vi "Specified_Channels_server.vi"(5 "Mode":T1, 6 "End time":dbl format="%.1f", 7 "Start time":dbl format="%.1f", 8 "Clients time":dbl, 9 "Requested channels":i32[](array[numeric])) -> (0 "Output array":dbl[][](array[numeric]) format="%.2f", 1 "Messages":string, 2 "Averaging Period":dbl[](array[numeric]) format="%.2f", 3 "Centre Times":dbl[](array[numeric]) format="%.1f", 4 "All Active Ch Names":string[](array[string]))   [LabVIEW 2021]
uses:
  ADAM Client/Sub VIs/ADAM Controls/Search_mode.ctl
  ADAM_Global.vi
  Sub VI's/Logged_Data_real_Global.vi
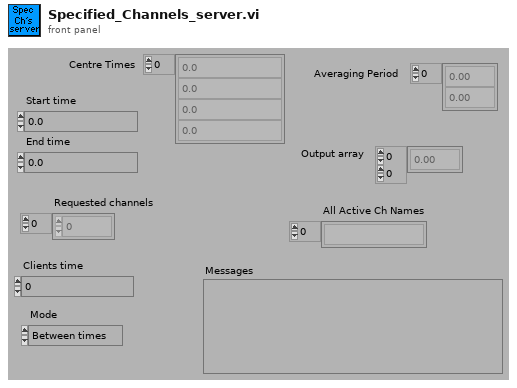
[diagram p1: front panel]
types:
  T1 = typedef "Search_mode.ctl" = enum16{"Between times", "All Times"}
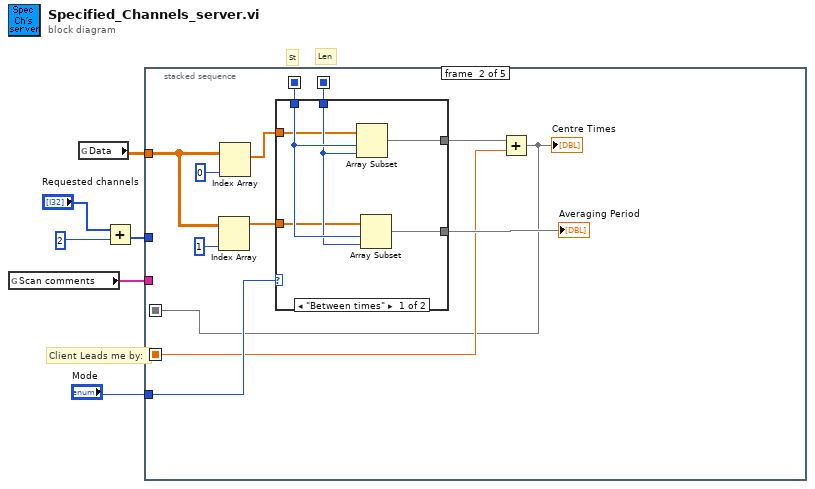
[diagram p0: block diagram]
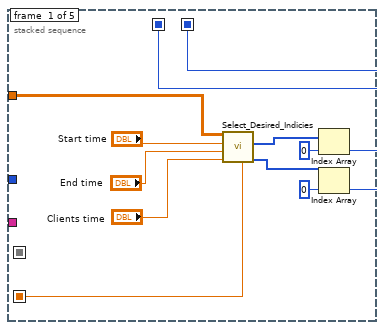
[diagram p2: hidden frame]
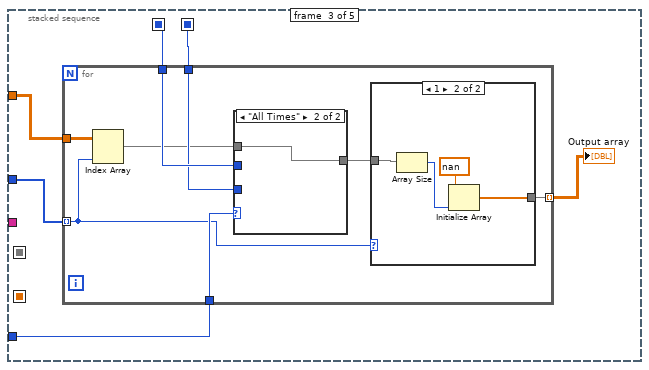
[diagram p4: hidden frame]
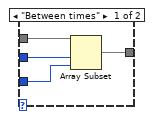
[diagram p6: hidden frame]
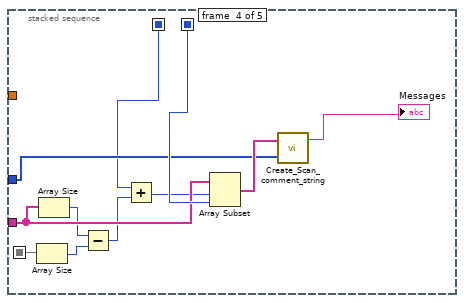
[diagram p7: hidden frame]
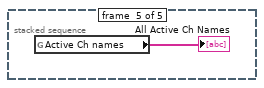
[diagram p8: hidden frame]
diagram:
  # "Len"
  # "St"
  # "Client Leads me by:"
  n1 = global read "ADAM_Global.vi" "Scan comments"() -> (w2:string[])
  n2 = global read "Logged_Data_real_Global.vi" "Data"() -> (w1:dbl[][])
  n3 = Add(x="Requested channels", y=2) -> (x+y=w4:i32[])
  n4 = stacked-sequence {
    seq-local: [w7 _ _ _ _] -> [_ w19 _ _ _]
    seq-local: [w10 _ _ _ _] -> [_ w26 w43 w65 _]
    seq-local: [w9 _ _ _ _] -> [_ w25 w42 w72 _]
    seq-local: [_ w18 _ _ _] -> [_ _ _ w63 _]
    tunnel: w1 -> [w14 w27 w41 _ _]
    tunnel: w4 -> [_ _ w40 w70 _]
    tunnel: w2 -> [_ _ _ w69 _]
    tunnel: "Mode" -> [_ w21 w39 _ _]
    frame #0 {
      n5 = call "Select_Desired_Indicies.vi"("Clients time"="Clients time", "End time"="End time", "Start time"="Start time", "Table values"=w14) -> ("Length"=w8:i32[], "Start integer"=w11:i32[], "Client leads me by:"=w7:dbl)  [unwired: 1 in, 3 out]
      n6 = Index Array(array=w11, index=0 ("Index")) -> (element=w10:i32)
      n7 = Index Array(array=w8, index=0 ("Index")) -> (element=w9:i32)
    }
    frame #1 {
      n8 = Index Array(array=w27, index (col)=1) -> (element=w24:dbl[])  [unwired: 1 in]
      n9 = Index Array(array=w27, index (col)=0) -> (element=w23:dbl[])  [unwired: 1 in]
      n10 = case shown="\"Between times\"" w21 {
        tunnel: [w35 w37] -> w20
        tunnel: w26 -> [w34 _]
        tunnel: w25 -> [w33 _]
        tunnel: w24 -> [w32 w36]
        tunnel: w23 -> [w31 w37]
        tunnel: [w30 w36] -> w22
        frame "Between times" {
          n11 = Array Subset(array=w31, index=w34, length=w33) -> (w35:dbl[])
          n12 = Array Subset(array=w32, index=w34, length=w33) -> (w30:dbl[])
        }
        frame "All Times" {
        }
      }
      "Averaging Period" <- w22
      n13 = Add(x=w20, y=w19) -> (x+y=w18:dbl[])
      "Centre Times" <- w18
    }
    frame #2 {
      n14 = for {
        tunnel: w42 -> [w49]
        tunnel: w43 -> [w50]
        tunnel: w40 -> [w46] mode=indexing
        tunnel: w41 -> [w51]
        tunnel: w39 -> [w48]
        tunnel: [w44] -> w38 mode=indexing
        n15 = Index Array(array=w51, index (col)=w46) -> (element=w47:dbl[])  [unwired: 1 in]
        n16 = case shown="\"All Times\"" w48 {
          tunnel: w47 -> [w60 w61]
          tunnel: [w59 w61] -> w45
          tunnel: w50 -> [w58 _]
          tunnel: w49 -> [w57 _]
          frame "Between times" {
            n17 = Array Subset(array=w60, index=w58, length=w57) -> (w59:dbl[])
          }
          frame "All Times" {
          }
        }
        n18 = case shown="1" w46 {
          tunnel: w45 -> [w52 w56]
          tunnel: [w52 w53] -> w44
          frame 2, Default {
          }
          frame 1 {
            n19 = Array Size(array=w56) -> (size(s)=w55:i32)
            n20 = Initialize Array(nan ("element"), w55) -> (w53:dbl[])
          }
        }
      }
      "Output array" <- w38
    }
    frame #3 {
      n21 = Array Size(array=w63) -> (size(s)=w67:i32)
      n22 = Array Size(array=w69) -> (size(s)=w68:i32)
      n23 = Subtract(x=w68, y=w67) -> (x-y=w66:i32)
      n24 = Add(x=w65, y=w66) -> (x+y=w64:i32)
      n25 = Array Subset(array=w69, index=w64, length=w72) -> (w71:string[])
      n26 = call "Create_Scan_comment_string.vi"("Requested channels"=w70, "Scan comments"=w71) -> ("Comment string"=→"Messages":string)
    }
    frame #4 {
      n27 = global read "ADAM_Global.vi" "Active Ch names"() -> (→"All Active Ch Names":string[])
    }
  }
